vi "test15.2-MappingRelationshipByLocalRegistration_WIthoutSubscriberName_State.vi"(8 "error in (no error)":errorcluster, 11 "TestCase in":refnum<class "testcase-CSMBroadcast.lvclass">) -> (0 "error out":errorcluster, 3 "TestCase out":refnum<class "testcase-CSMBroadcast.lvclass">)   [LabVIEW 2017, in "testcase-CSMBroadcast.lvclass"]
uses:
  testcase-CSMBroadcast.lvclass
  47fe1622-87c8-40c1-b9cf-9bbb5cd90bb5.vi
  <vilib>/addons/_JKI Toolkits/VI Tester/TestCase.llb/TestCase.lvclass
  src/user.lib/_NEVSTOP/Communicable State Machine(CSM)/Communicable State Machine.lvlib
  CSM/CSM-Testcase.lvlib
  C:/Program Files (x86)/National Instruments/LabVIEW 2017/vi.lib/addons/_JKI Toolkits/VI Tester/TestCase.llb/TestCase.lvclass
panel:
  out "Loop Count":i32
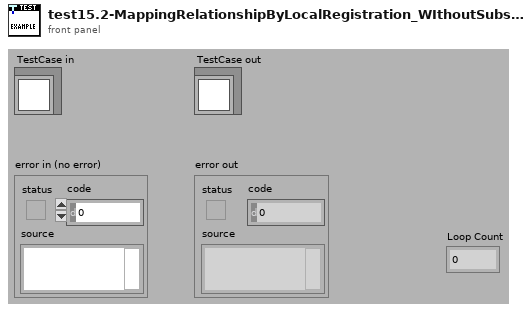
[diagram p1: front panel]
types:
  T1 = cluster{"Status":string, "Source CSM":string, "Target CSM":string, "Target API":string}[]
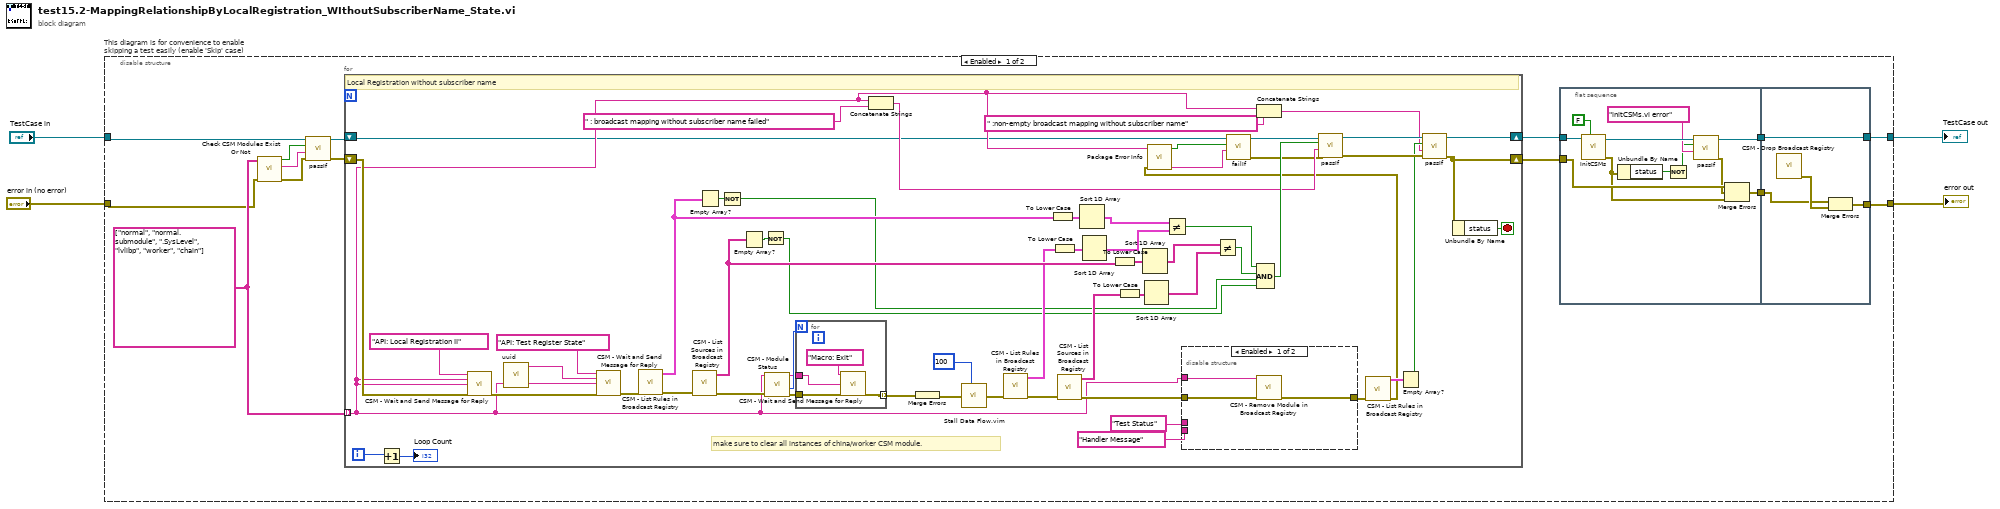
[diagram p0: block diagram]
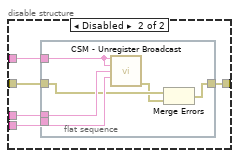
[diagram p2: hidden frame]
diagram:
  n1 = disable-structure "This diagram is for convenience to enable skipping a test easily (enable 'Skip' case)" shown="Enabled" {
    disable-tunnel: "TestCase in" -> [w14 w114]
    disable-tunnel: [w8 w112] -> w1
    disable-tunnel: [w7 w113] -> w3
    disable-tunnel: "error in (no error)" -> [w13 w111]
    frame Enabled {
      w15 = string[] ["normal", "normal.submodule", ".SysLevel", "lvlibp", "worker", "chain"]
      n2 = call "Check CSM Modules Exist Or Not.vi"("error in"=w13, "CSM names in"=w15) -> ("error out"=w16:errorcluster, "Debug string"=w17:string, "All Modules Exist?"=w18:bool)  [unwired: 7 in]
      n3 = call-dynamic "passIf.vi"("error in (no error)"=w16, "message (\"\")"=w17, "pass"=w18, "TestCase in"=w14) -> ("error out"=w5:errorcluster, "TestCase out"=w6:refnum<class "testcase-CSMBroadcast.lvclass">)  [unwired: 6 in]
      n4 = for {
        tunnel: w15 -> [w37] mode=indexing
        shift-right: [w56] -> w10
        shift-left: w6 -> [w35]
        shift-right: [w58] -> w9
        shift-left: w5 -> [w52]
        i -> [w79]
        stop <- w86 stop-if-true
        # "make sure to clear all instances of china/worker CSM module."
        # "Local Registration without subscriber name"
        n5 = Increment(x=w79) -> (x+1=→"Loop Count":i32)
        n6 = call "CSM - Wait and Send Message for Reply.vi"("State"="API: Local Registration II", "Arguments (\"\")"=w37, "Target Module"=w37, "Error In (No Error)"=w52) -> ("error out"=w91:errorcluster)  [unwired: 8 in, 3 out]
        n7 = call "uuid.vi"() -> ("UUID"=w89:string)  [unwired: 11 in]
        n8 = call "CSM - Wait and Send Message for Reply.vi"("State"="API: Test Register State", "Arguments (\"\")"=w89, "Target Module"=w37, "Error In (No Error)"=w91) -> ("error out"=w88:errorcluster)  [unwired: 8 in, 3 out]
        n9 = call "CSM - List Rules in Broadcast Registry.vi"("error in (no error)"=w88) -> ("error out"=w85:errorcluster, "Rule Entries"=w77:T1)  [unwired: 8 in, 1 out]
        n10 = call "CSM - List Sources in Broadcast Registry.vi"("error in (no error)"=w85) -> ("error out"=w49:errorcluster, "Broadcast Names"=w74:string[])  [unwired: 9 in]
        n11 = Empty Array?(array=w77) -> (empty?=w76:bool)
        n12 = Not(x=w76) -> (.not. x?=w71:bool)
        n13 = Empty Array?(array=w74) -> (empty?=w75:bool)
        n14 = Not(x=w75) -> (.not. x?=w70:bool)
        n15 = call "CSM - Module Status.vi"("Error In"=w49, "CSM Name"=w37) -> ("error out"=w48:errorcluster, "#Nodes"=w51:i32, "CSM Name (Dup)"=w50:string)  [unwired: 5 in, 2 out]
        n16 = for {
          N: w51 -> [_]
          tunnel: [w95] -> w87 mode=indexing
          tunnel: w50 -> [w94]
          tunnel: w48 -> [w93]
          n17 = call "CSM - Wait and Send Message for Reply.vi"("State"="Macro: Exit", "Target Module"=w94, "Error In (No Error)"=w93) -> ("error out"=w95:errorcluster)  [unwired: 9 in, 3 out]
        }
        n18 = Concatenate Strings(w37, " : broadcast mapping without subscriber name failed" ("string")) -> (w44:string)
        n19 = Merge Errors(w87) -> (w43:errorcluster)
        n20 = call "Stall Data Flow.vim"("value in"=w43, "milliseconds to wait"=u32 100) -> ("value out"=w42:errorcluster)  [unwired: 1 out]
        n21 = call "CSM - List Rules in Broadcast Registry.vi"("error in (no error)"=w42) -> ("error out"=w84:errorcluster, "Rule Entries"=w73:T1)  [unwired: 8 in, 1 out]
        n22 = To Lower Case(string=w77) -> (all lower case string=w83:T1)
        n23 = To Lower Case(string=w73) -> (all lower case string=w82:T1)
        n24 = call "CSM - List Sources in Broadcast Registry.vi"("error in (no error)"=w84) -> ("error out"=w68:errorcluster, "Broadcast Names"=w72:string[])  [unwired: 9 in]
        n25 = Sort 1D Array(array=w83) -> (sorted array=w65:T1)
        n26 = Sort 1D Array(array=w82) -> (sorted array=w64:T1)
        n27 = To Lower Case(string=w74) -> (all lower case string=w81:string[])
        n28 = To Lower Case(string=w72) -> (all lower case string=w80:string[])
        n29 = Sort 1D Array(array=w81) -> (sorted array=w62:string[])
        n30 = Sort 1D Array(array=w80) -> (sorted array=w61:string[])
        n31 = Not Equal?(x=w65, y=w64) -> (x != y?=w63:bool)
        n32 = disable-structure shown="Enabled" {
          disable-tunnel: w68 -> [w99 w101]
          disable-tunnel: [w98 w100] -> w55
          disable-tunnel: w37 -> [w97 w102]
          disable-tunnel: "Test Status" ("Status") -> [_ w104]
          disable-tunnel: "Handler Message" ("Response Message (If \"\", Same as Source Message)") -> [_ w103]
          frame Enabled {
            n33 = call "CSM - Remove Module in Broadcast Registry.vi"("CSM Name"=w97, "Error In"=w99) -> ("error out"=w98:errorcluster)  [unwired: 12 in, 1 out]
          }
          frame Disabled {
            n34 = flat-sequence {
              tunnel: w104 -> [w110]
              tunnel: w103 -> [w109]
              tunnel: w102 -> [w108]
              tunnel: w101 -> [w107]
              tunnel: [w105] -> w100
              frame #0 {
                n35 = call "CSM - Unregister Broadcast.vi"("CSM Name(Empty for Broadcast Event)"=w108, "Source CSM Name (* as Default)"=w108, "Trigger"=w110, "API (\"*\" as Default)"=w109) -> ("error out"=w106:errorcluster)  [unwired: 10 in, 1 out]
                n36 = Merge Errors(w107, w106) -> (w105:errorcluster)
              }
            }
          }
        }
        n37 = Not Equal?(x=w62, y=w61) -> (x != y?=w60:bool)
        n38 = Concatenate Strings(w37, " :non-empty broadcast mapping without subscriber name" ("string")) -> (w45:string)
        n39 = Compound Arithmetic op=AND(w63, w60, w71, w70) -> (w69:bool)
        n40 = call "CSM - List Rules in Broadcast Registry.vi"("error in (no error)"=w55) -> ("error out"=w38:errorcluster, "Rule Entries"=w54:T1)  [unwired: 8 in, 1 out]
        n41 = call "Package Error Info.vi"("error in"=w38, "String in"=w37) -> ("packed error info out"=w40:string, "error status"=w39:bool)  [unwired: 8 in]
        n42 = call-dynamic "failIf.vi"("message (\"\")"=w40, "fail"=w39, "TestCase in"=w35) -> ("error out"=w36:errorcluster, "TestCase out"=w34:refnum<class "testcase-CSMBroadcast.lvclass">)  [unwired: 7 in]
        n43 = call-dynamic "passIf.vi"("error in (no error)"=w36, "message (\"\")"=w44, "pass"=w69, "TestCase in"=w34) -> ("error out"=w59:errorcluster, "TestCase out"=w57:refnum<class "testcase-CSMBroadcast.lvclass">)  [unwired: 6 in]
        n44 = Empty Array?(array=w54) -> (empty?=w53:bool)
        n45 = call-dynamic "passIf.vi"("error in (no error)"=w59, "message (\"\")"=w45, "pass"=w53, "TestCase in"=w57) -> ("error out"=w58:errorcluster, "TestCase out"=w56:refnum<class "testcase-CSMBroadcast.lvclass">)  [unwired: 6 in]
        n46 = Unbundle By Name(w58) -> ("status"=w86:bool)
      }
      n47 = flat-sequence {
        tunnel: w10 -> [w29]
        tunnel: [w26] -> w12
        tunnel: w9 -> [w23]
        tunnel: [w20] -> w11
        tunnel: w12 -> [w32]
        tunnel: [w32] -> w8
        tunnel: [w31] -> w7
        tunnel: w11 -> [w30]
        frame #0 {
          n48 = call "InitCSMs.vi"("Enable building lvlibp?"=FALSE, "testcase-CSMStatus in"=w29) -> ("error out"=w21:errorcluster, "testcase-CSMStatus out"=w27:refnum<class "testcase-CSMBroadcast.lvclass">)  [unwired: 8 in]
          n49 = Unbundle By Name(w21) -> ("status"=w25:bool)
          n50 = Not(x=w25) -> (.not. x?=w19:bool)
          n51 = call-dynamic "passIf.vi"("message (\"\")"="initCSMs.vi error" ("message (\"\")"), "pass"=w19, "TestCase in"=w27) -> ("error out"=w22:errorcluster, "TestCase out"=w26:refnum<class "testcase-CSMBroadcast.lvclass">)  [unwired: 7 in]
          n52 = Merge Errors(w23, w22, w21) -> (w20:errorcluster)
        }
        frame #1 {
          n53 = call "CSM - Drop Broadcast Registry.vi"() -> ("error out"=w33:errorcluster)  [unwired: 15 in]
          n54 = Merge Errors(w30, w33) -> (w31:errorcluster)
        }
      }
    }
    frame Disabled {
      # "skip test result while test is under development"
      n55 = call <vilib>:"skip.vi"("error in (no error)"=w111, "TestCase in"=w114) -> ("error out"=w113:errorcluster, "TestCase out"=w112:refnum<class "testcase-CSMBroadcast.lvclass">)  [unwired: 8 in]
    }
  }
  "error out" <- w3
  "TestCase out" <- w1
